vi "Actor Core.vi"(8 "error in":errorcluster, 11 "Node Guard in":refnum<class "Node Guard.lvclass">) -> (0 "error out":errorcluster, 3 "Actor out":refnum<class "Actor.lvclass">)   [LabVIEW 2020, in "CANopen.lvlib" / "Network Management.lvlib" / "Node Guard.lvlib" / "Node Guard.lvclass"]
doc: "<p>(<strong>Filename</strong>: <span class=\"dnl\">Actor Framework.lvlib:Actor.lvclass:Actor Core.vi</span>)</p>\n<p>Receives messages to the actor, reacts to them, and initiates any error handling that may shut the actor down.</p>\n<p>Descendant classes may override this VI to append parallel tasks for the actor to complete while it handles messages. Overrides use the <a href=\"nihelplauncher://docs/csh?context=lvcore_glang_udclass\">Call Parent Class Method</a> node.</p>"
uses:
  Node Guard.lvclass
  Node Guard.lvclass/Node Guard.ctl
  C:/Program Files/National Instruments/LabVIEW 2026/vi.lib/ActorFramework/Actor/Actor.lvclass
  D:/git/CANopen-LabVIEW/source/Network Management/Node Guard/Node Guard.lvclass
  Logging/Log Level.vi
  Logging/CANopen Logging.lvlib
  HAL/Source/Interfaces/ICAN CC Frame/ICAN CC Frame.lvclass
  <vilib>/ActorFramework/Actor/Actor.lvclass
  Node Guard Messages/Update Node State Msg/Update Node State Msg.lvclass
  HAL/Source/Interfaces/ICommunicate/ICommunicate.lvclass
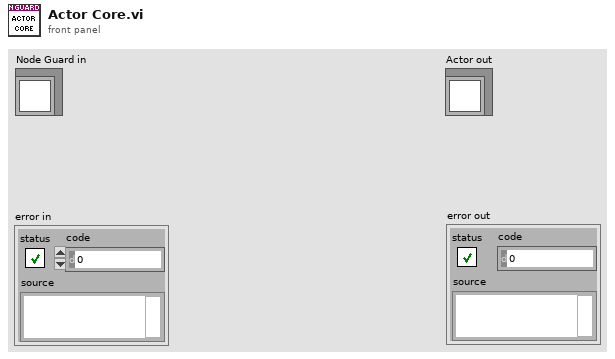
[diagram p1: front panel]
types:
  T1 = enum16{"Error", "Warn", "Info", "Debug", "Trace"}
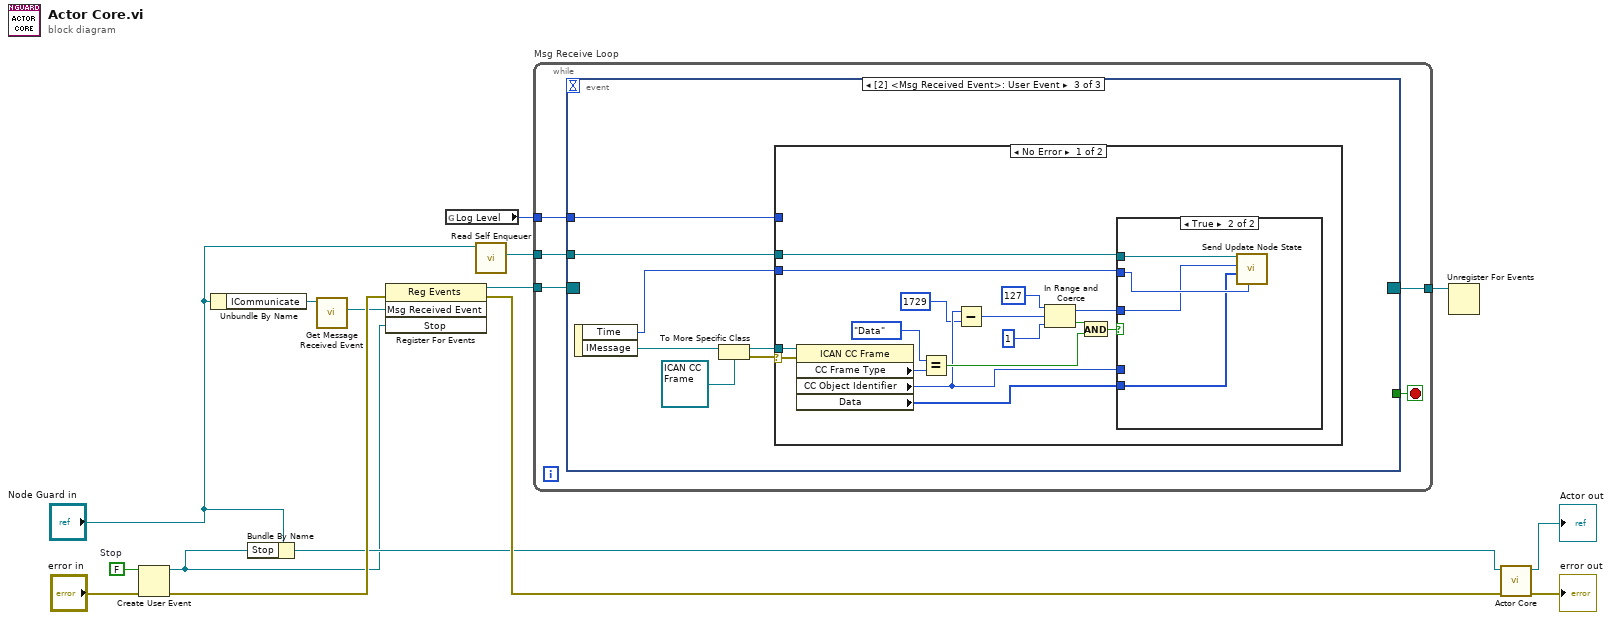
[diagram p0: block diagram]
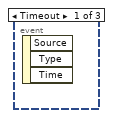
[diagram p2: hidden frame]
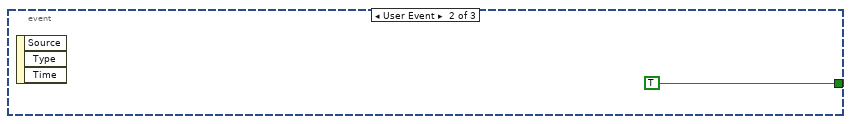
[diagram p3: hidden frame]
diagram:
  w12 = FALSE  # Stop
  n1 = Create User Event(user event datatype=w12, error in="error in") -> (user event=w4:refnum<user-event>, error out=w15:errorcluster)
  n2 = Unbundle By Name("Node Guard in") -> ("ICommunicate"=w11:refnum<class "ICommunicate.lvclass">)
  n3 = Bundle By Name(cluster="Node Guard in", "Stop"=w4) -> (w5:refnum<class "Node Guard.lvclass">)
  n4 = call-dynamic "Get Message Received Event.vi"("ICommunicate in"=w11) -> ("Msg Received Event"=w1:refnum<user-event>)  [unwired: 8 in, 2 out]
  n5 = register-events(error in=w15, w1, w4) -> (reference out=w8:refnum<event-registration>, error out=w9:errorcluster)  [unwired: 1 in]
  n6 = global read "Log Level.vi" "Log Level"() -> (w7:T1)
  n7 = call <vilib>:"Read Self Enqueuer.vi"("Actor"="Node Guard in") -> ("Self Enqueuer"=w3:refnum<class "Message Enqueuer.lvclass">)  [unwired: 10 in]
  n8 = while "Msg Receive Loop" {
    tunnel: w8 -> [w19]
    tunnel: [w18] -> w10
    tunnel: w3 -> [w17]
    tunnel: w7 -> [w16]
    stop <- w20 stop-if-true
    n9 = event shown="[2] <Msg Received Event>: User Event" {
      selector: w19 -> [_ _ _]
      dyn-events: [_ _ _] -> w18
      timeout: _ -> [_ _ _]
      tunnel: [_ TRUE _] -> w20
      tunnel: w17 -> [_ _ w23]
      tunnel: w16 -> [_ _ w27]
      event Timeout {
        n10 = event-data() -> ()  [unwired: 1 in, 3 out]
      }
      event User Event {
        n11 = event-data() -> ()  [unwired: 1 in, 3 out]
      }
      event User Event {
        n12 = event-data() -> ("Time"=w22:u32, "IMessage"=w28:refnum<class "IMessage.lvclass">)  [unwired: 1 in]
        n13 = To More Specific Class(target class=refnum<class "ICAN CC Frame.lvclass"> refnum ("ICAN CC Frame"), reference=w28) -> (specific class reference=w26:refnum<class "ICAN CC Frame.lvclass">, error out=w24:errorcluster)  [unwired: 1 in]
        n14 = case shown="No Error" w24 {
          selector: w24 -> [w44 _]
          tunnel: w26 -> [w43 _]
          tunnel: w27 -> [_ _]
          tunnel: w23 -> [w39 _]
          tunnel: w22 -> [w38 _]
          frame No Error {
            n15 = property class="ICAN CC Frame"(reference=w43, error in=w44) -> ("CC Frame Type"=w37:enum8{"Data", "Remote", "Error", "Overload"}, "CC Object Identifier"=w31:u32, "Data"=w40:u8[])  [unwired: 2 out]
            n16 = Equal?(x=enum8{"Data", "Remote", "Error", "Overload"}."Data", y=w37) -> (x = y?=w33:bool)
            n17 = Subtract(x=w31, y=u32 1729) -> (x-y=w29:u32)
            n18 = In Range and Coerce(upper limit=u32 127, x=w29, lower limit=u32 1) -> (coerced(x)=w32:u32, In Range?=w34:bool)
            n19 = And(x=w34, y=w33) -> (x .and. y?=w35:bool)
            n20 = case shown="True" w35 {
              tunnel: w40 -> [_ w46]
              tunnel: w39 -> [_ w48]
              tunnel: w31 -> [_ _]
              tunnel: w38 -> [_ w47]
              tunnel: w32 -> [_ w45]
              frame False {
              }
              frame True {
                n21 = call "Send Update Node State.vi"("Received Tick"=w47, "Frame Data"=w46, "Node ID"=w45, "Message Enqueuer"=w48) -> ()  [unwired: 6 in, 2 out]
              }
            }
          }
          frame Error {
          }
        }
      }
    }
  }
  n22 = Unregister For Events(event registration refnum=w10) -> ()  [unwired: 1 in, 1 out]
  n23 = call-parent "Actor Core.vi"("error in"=w9, "Actor in"=w5) -> ("error out"=→"error out":errorcluster, "Actor out"=→"Actor out":refnum<class "Actor.lvclass">)  [unwired: 8 in]
